vi "Cast.vi"(8 "error in (no error)":errorcluster, 10 "Cast Type":refnum<class "Basic Type.lvclass">, 11 "Basic Type in":refnum<class "Basic Type.lvclass">) -> (0 "error out":errorcluster, 3 "Basic Type out":refnum<class "Basic Type.lvclass">)   [LabVIEW 2020, in "Protobuf RAW.lvlib" / "Basic Type.lvclass"]
uses:
  Basic Type.lvclass
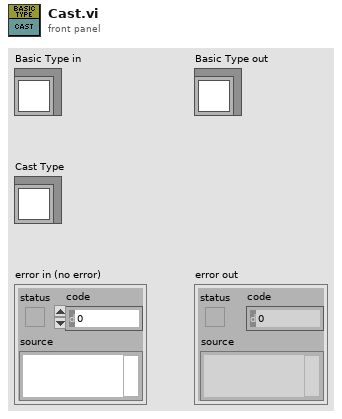
[diagram p1: front panel]
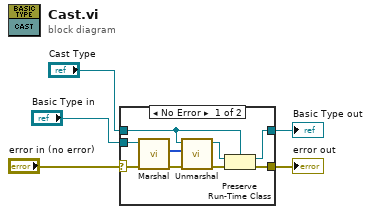
[diagram p0: block diagram]
diagram:
  n1 = case shown="No Error" "error in (no error)" {
    selector: "error in (no error)" -> [w13 w16]
    tunnel: [w6 w16] -> w4
    tunnel: [w7 w15] -> w2
    tunnel: "Basic Type in" -> [w14 _]
    tunnel: "Cast Type" -> [w9 w15]
    frame No Error {
      n2 = call-dynamic "Marshal.vi"("error in (no error)"=w13, "Tag in"=w14) -> ("error out"=w11:errorcluster, "Buffer"=w12:u8[])  [unwired: 7 in, 1 out]
      n3 = call-dynamic "Unmarshal.vi"("error in (no error)"=w11, "Buffer"=w12, "Tag in"=w9) -> ("error out"=w8:errorcluster, "Tag out"=w10:refnum<class "Basic Type.lvclass">)  [unwired: 6 in, 1 out]
      n4 = Preserve Run-Time Class(object in=w10, error in=w8, 2:w9) -> (object out=w7:refnum<class "Basic Type.lvclass">, error out=w6:errorcluster)
    }
    frame Error {
    }
  }
  "error out" <- w4
  "Basic Type out" <- w2
